vi "EmergencyCooler.vi"(5 "Day of Year":u32, 6 "Unique Object Identifier":string, 7 "Day Time":u32, 8 "Error In":errorcluster, 10 "Energy flow IN":T5, 11 "DataFlowIN":T4) -> (0 "Error Out":errorcluster, 1 "Emergency cooling":bool, 2 "Energy flow OUT":T5, 3 "DataFlowOUT":T4)   [LabVIEW 2017]
uses:
  classes/DataCollector.lvclass
  classes/DataHandler.lvclass
  classes/SimulationParameter.lvclass
panel:
  out "Simulation Parameter":T1
  in  "Operating Parameter":T2
  out "Control Parameter":T3
  out "List of Fieldelements":string[](array[string])
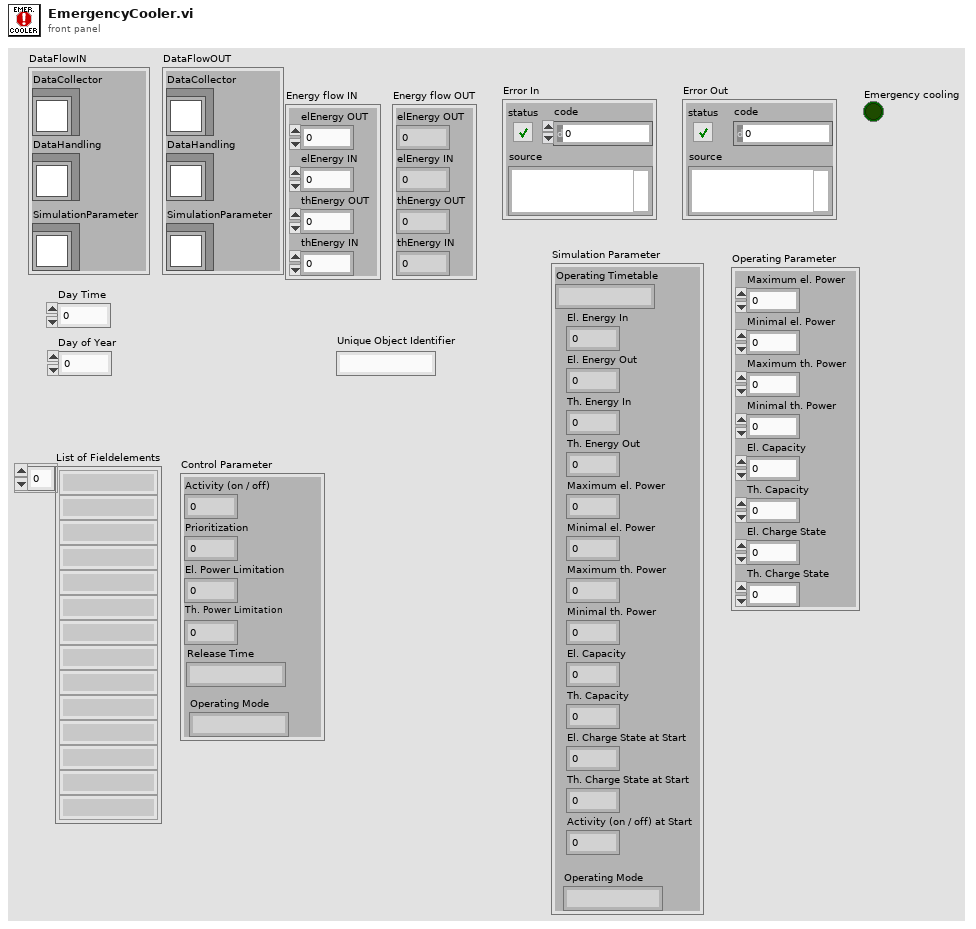
[diagram p1: front panel]
types:
  T1 = cluster{"Operating Timetable":string, "El. Energy In":dbl, "El. Energy Out":dbl, "Th. Energy In":dbl, "Th. Energy Out":dbl, "Maximum el. Power":dbl, "Minimal el. Power":dbl, "Maximum th. Power":dbl, "Minimal th. Power":dbl, "El. Capacity":dbl, "Th. Capacity":dbl, "El. Charge State at Start":dbl, "Th. Charge State at Start":dbl, "Activity (on / off) at Start":i64, "Operating Mode":string}
  T2 = cluster{"Maximum el. Power":dbl, "Minimal el. Power":dbl, "Maximum th. Power":dbl, "Minimal th. Power":dbl, "El. Capacity":dbl, "Th. Capacity":dbl, "El. Charge State":dbl, "Th. Charge State":dbl}
  T3 = cluster{"Activity (on / off)":i64, "Prioritization":i64, "El. Power Limitation":dbl, "Th. Power Limitation":dbl, "Release Time":string, "Operating Mode":string}
  T4 = cluster{"DataCollector":refnum<class "DataCollector.lvclass">, "DataHandling":refnum<class "DataHandler.lvclass">, "SimulationParameter":refnum<class "SimulationParameter.lvclass">}
  T5 = cluster{"elEnergy OUT":dbl, "elEnergy IN":dbl, "thEnergy OUT":dbl, "thEnergy IN":dbl}
  T6 = cluster{"elEnergy OUT":dbl, "thEnergy OUT":dbl, "thEnergy IN":dbl, "thEnergy IN":dbl}
  T7 = cluster{"Day Time":u32, "Day of Year":u32, cluster{"elEnergy OUT":dbl, "thEnergy OUT":dbl, "thEnergy IN":dbl, "thEnergy IN":dbl}, "Operating Parameter":cluster{"Maximum el. Power":dbl, "Minimal el. Power":dbl, "Maximum th. Power":dbl, "Minimal th. Power":dbl, "El. Capacity":dbl, "Th. Capacity":dbl, "El. Charge State":dbl, "Th. Charge State":dbl}, "Control Parameter":cluster{"Activity (on / off)":i64, "Prioritization":i64, "El. Power Limitation":dbl, "Th. Power Limitation":dbl, "Release Time":string, "Operating Mode":string}}
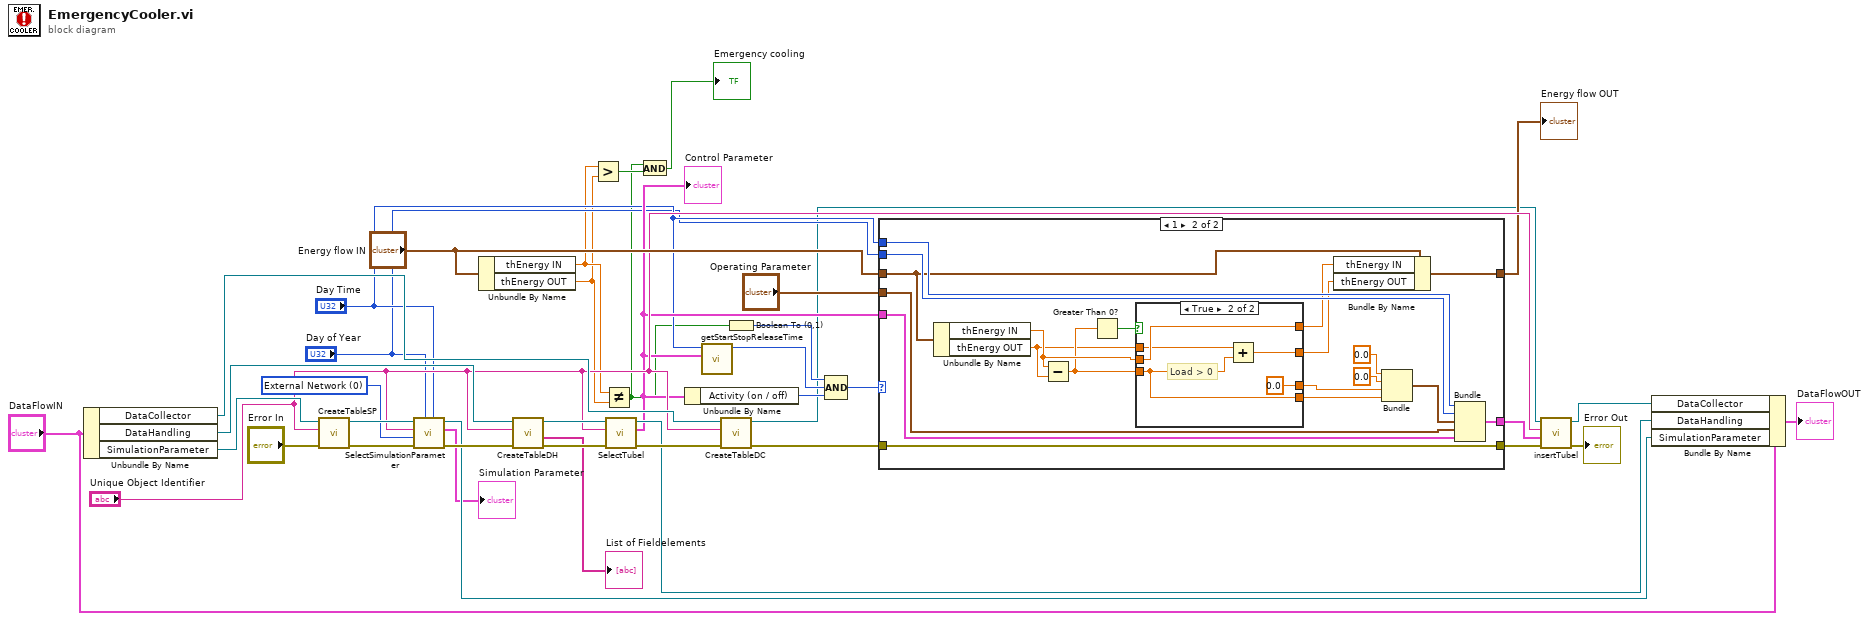
[diagram p0: block diagram]
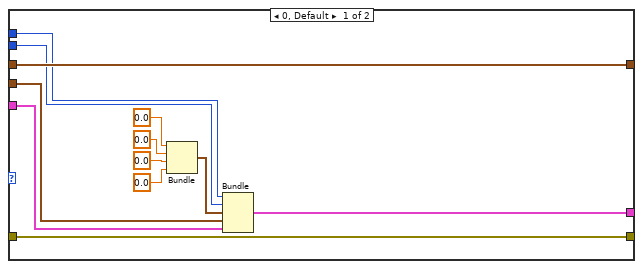
[diagram p2: hidden frame]
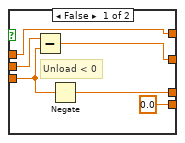
[diagram p3: hidden frame]
diagram:
  w21 = u16 0 items=["External Network", "Consumer", "Producer", "Sorage"] ("Type of Simulation")
  n1 = Unbundle By Name("DataFlowIN") -> ("DataCollector"=w39:refnum<class "DataCollector.lvclass">, "DataHandling"=w34:refnum<class "DataHandler.lvclass">, "SimulationParameter"=w29:refnum<class "SimulationParameter.lvclass">)
  n2 = call-dynamic "CreateTableSP.vi"("error in (no error)"="Error In", "Name of Table"="Unique Object Identifier", "SimulationParameter in"=w29) -> ("error out"=w32:errorcluster, "SimulationParameter out"=w31:refnum<class "SimulationParameter.lvclass">)  [unwired: 5 in, 2 out]
  n3 = call-dynamic "SelectSimulationParameter.vi"("Day of Year"="Day Time", "Day Time"="Day of Year", "error in (no error)"=w32, "Type of Simulation"=w21, "Unique Object Identifier"="Unique Object Identifier", "SimulationParameter in"=w31) -> ("error out"=w30:errorcluster, "Cluster"=→"Simulation Parameter":T1, "SimulationParameter out"=w28:refnum<class "SimulationParameter.lvclass">)  [unwired: 3 in]
  n4 = Unbundle By Name("Energy flow IN") -> ("thEnergy IN"=w2:dbl, "thEnergy OUT"=w1:dbl)
  n5 = call-dynamic "CreateTableDH.vi"("error in (no error)"=w30, "Name of Table"="Unique Object Identifier", "DataHandler in"=w34) -> ("error out"=w37:errorcluster, "List of Fieldelements"=→"List of Fieldelements":string[], "DataHandler out"=w35:refnum<class "DataHandler.lvclass">)  [unwired: 5 in, 1 out]
  n6 = Greater?(x=w2, y=w1) -> (0:w5:bool)
  n7 = Not Equal?(x=w2, y=w1) -> (x != y?=w4:bool)
  n8 = call-dynamic "SelectTubel.vi"("error in (no error)"=w37, "Unique Object Identifier"="Unique Object Identifier", "DataHandler in"=w35) -> ("error out"=w36:errorcluster, "Control Parameter"=w16:T3, "DataHandler out"=w33:refnum<class "DataHandler.lvclass">)  [unwired: 5 in, 1 out]
  "Control Parameter" <- w16
  n9 = And(x=w4, y=w5) -> (x .and. y?=→"Emergency cooling":bool)
  n10 = Unbundle By Name(w16) -> ("Activity (on / off)"=w23:i64)
  n11 = call "getStartStopReleaseTime.vi"("Control Parameter"=w16, "Day Time"="Day Time") -> ("Activity (on / off)"=w24:i64)  [unwired: 9 in]
  n12 = call "CreateTableDC.vi"("error in (no error)"=w36, "Name of Table"="Unique Object Identifier", "DataCollector in"=w39) -> ("error out"=w6:errorcluster, "DataCollector out"=w7:refnum<class "DataCollector.lvclass">)  [unwired: 7 in]
  n13 = Boolean To (0,1)(Boolean=w4) -> (0, 1=w25:i16)
  n14 = Compound Arithmetic op=AND(w25, w24, w23) -> (w22:i64)
  n15 = case shown="1" w22 {
    tunnel: w6 -> [w50 w53]
    tunnel: [w50 w53] -> w27
    tunnel: "Day Time" -> [w43 w70]
    tunnel: "Day of Year" -> [w42 w69]
    tunnel: "Operating Parameter" -> [w45 w54]
    tunnel: "Energy flow IN" -> [w51 w68]
    tunnel: [w51 w67] -> w9
    tunnel: w16 -> [w40 w65]
    tunnel: [w41 w62] -> w26
    frame 0, Default {
      n16 = Bundle("elEnergy OUT"=0.0, "thEnergy OUT"=0.0, "thEnergy IN"=0.0, "thEnergy IN"=0.0) -> (w44:T6)  [unwired: 1 in]
      n17 = Bundle("Day Time"=w43, "Day of Year"=w42, w44, "Operating Parameter"=w45, "Control Parameter"=w40) -> (w41:T7)  [unwired: 1 in]
    }
    frame 1 {
      n18 = Unbundle By Name(w68) -> ("thEnergy IN"=w61:dbl, "thEnergy OUT"=w59:dbl)
      n19 = Subtract(x=w61, y=w59) -> (x-y=w60:dbl)
      n20 = Greater Than 0?(x=w60) -> (x > 0?=w52:bool)
      n21 = case shown="True" w52 {
        tunnel: w61 -> [w76 w81]
        tunnel: w60 -> [w72 w77]
        tunnel: w59 -> [w75 w80]
        tunnel: [w75 w81] -> w58
        tunnel: [w74 w78] -> w57
        tunnel: [w71 0.0 ("thEnergy IN")] -> w56
        tunnel: [0.0 ("thEnergy IN") w77] -> w55
        frame False {
          # "Unload < 0"
          n22 = Subtract(x=w76, y=w72) -> (x-y=w74:dbl)
          n23 = Negate(x=w72) -> (-x=w71:dbl)
        }
        frame True {
          # "Load > 0"
          n24 = Add(x=w80, y=w77) -> (x+y=w78:dbl)
        }
      }
      n25 = Bundle By Name(cluster=w68, "thEnergy IN"=w58, "thEnergy OUT"=w57) -> (w67:T5)
      n26 = Bundle("elEnergy OUT"=0.0, "thEnergy OUT"=0.0, "thEnergy IN"=w56, "thEnergy IN"=w55) -> (w66:T6)  [unwired: 1 in]
      n27 = Bundle("Day Time"=w70, "Day of Year"=w69, w66, "Operating Parameter"=w54, "Control Parameter"=w65) -> (w62:T7)  [unwired: 1 in]
    }
  }
  "Energy flow OUT" <- w9
  n28 = call-dynamic "insertTubel.vi"("error in (no error)"=w27, "Data Cluster"=w26, "Name of Table"="Unique Object Identifier", "DataCollector in"=w7) -> ("error out"=→"Error Out":errorcluster, "DataCollector out"=w38:refnum<class "DataCollector.lvclass">)  [unwired: 6 in]
  n29 = Bundle By Name(cluster="DataFlowIN", "DataCollector"=w38, "DataHandling"=w33, "SimulationParameter"=w28) -> (→"DataFlowOUT":T4)
